vi "Machs.vi"(0 "Heizen?Mach1":bool, 1 "Heizen?Mach2":bool, 2 "PIDMach1":T1 {"proportional gain (Kc)" format="%.11g"; "integral gain (Kc*Ts/Ti)" format="%.11g"; "derivative gain (Kc*Td/Ts)" format="%.11g"}, 3 "PIDMach2":T1 {"proportional gain (Kc)" format="%.11g"; "integral gain (Kc*Ts/Ti)" format="%.11g"; "derivative gain (Kc*Td/Ts)" format="%.11g"}, 4 "Umax[V]Mach1":fxp<+/-,16,4> format="%.14g", 5 "Umax[V]Mach2":fxp<+/-,16,4> format="%.14g", 6 "USetp[V]Mach1":fxp<+/-,16,4> format="%.14g", 7 "USetp[V]Mach2":fxp<+/-,16,4> format="%.14g", 10 "Per[us]Mach":u16 caption="Periode Mach [us]", 11 "Mach1maxHigh":u16, 12 "vor der Messung [us]Mach":u16=200, 14 "wie viele Messwerte?Mach":u16, 15 "Mach2High?":bool, 16 "Abstand zwischen Messungen [us]Mach":u16 caption="Abstand zwischen Messungen Mach [us]", 17 "Mach2High":u16) -> (20 "U[V]Mach1":fxp<+/-,16,4> format="%.25g", 21 "U[V]Mach2":fxp<+/-,16,4> format="%.25g", 23 "Mach1maxHigh":u16, 26 "Mach2High?":bool, 27 "Mach2High":u16)   [LabVIEW 2010]
uses:
  <vilib>/eio/EIONode/EIONode.xnode
  <vilib>/rvi/eio/nirviEIOImplementation/nirviEIOImplementation.xnode
  <vilib>/rvi/eio/common/nirviEmuClasses.ctl
  <vilib>/rvi/FXPMathLib/FxpAdd/XNode/nifxpmath_Add.xnode
  <vilib>/rvi/FXPMathLib/FxpAdd/subVIs/nifxpmath_Add_SimConfig.ctl
  <vilib>/fxp/LVFixedPointQuantizationPolicyTypeDef.ctl
  <vilib>/fxp/LVFixedPointOverflowPolicyTypeDef.ctl
  <vilib>/rvi/FXPMathLib/FxpDiv/XNode/nifxpmath_Div.xnode
  <vilib>/rvi/FXPMathLib/FxpDiv/subVIs/nifxpmath_Div_SimConfig.ctl
  <vilib>/rvi/FXPMathLib/FxpMul/XNode/nifxpmath_Multiplier.xnode
  <vilib>/rvi/FXPMathLib/FxpMul/subVIs/nifxpmath_Mul_SimConfig.ctl
  <vilib>/rvi/FXPMathLib/FxpSqrt/XNode/nifxpmath_Sqrt.xnode
  <vilib>/rvi/FXPMathLib/FxpSqrt/subVIs/nifxpmath_Sqrt_SimConfig.ctl
  <vilib>/rvi/FXPMathLib/FxpConvert/XNode/nifxpmath_Convert.xnode
  <vilib>/rvi/FXPMathLib/FxpConvert/subVIs/nifxpmath_Convert_SimConfig.ctl
  <vilib>/addons/control/pid/fpga.llb/XNode/niFpgaPID.xnode
  <vilib>/rvi/eio/common/nirviEmuTemplateMethod_noerrors.vi
  <vilib>/rvi/FXPMathLib/FxpAdd/simVIs/DllFxpAddTemp_sub.vi
  <vilib>/rvi/FXPMathLib/FxpDiv/simVIs/DllFxpDivTemp_sub.vi
  <vilib>/rvi/FXPMathLib/FxpMul/simVIs/DllFxpMulTemp_sub.vi
  <vilib>/rvi/FXPMathLib/FxpSqrt/simVIs/DllSqrtTemp_sub.vi
  <vilib>/rvi/FXPMathLib/FxpConvert/simVIs/DllFxpConvertTemp_sub.vi
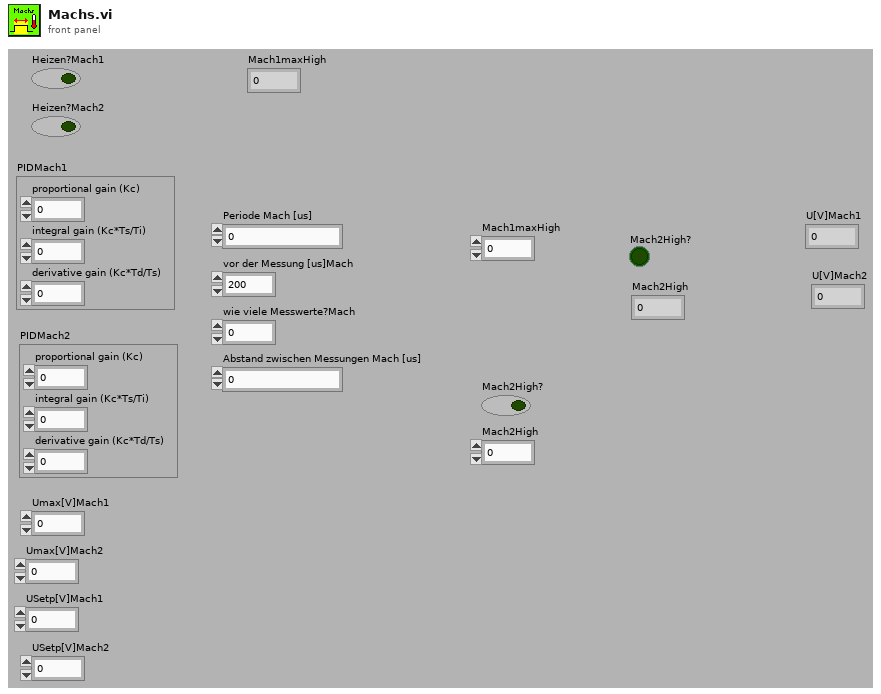
[diagram p1: front panel]
types:
  T1 = cluster{"proportional gain (Kc)":fxp<+/-,16,8>, "integral gain (Kc*Ts/Ti)":fxp<+/-,16,8>, "derivative gain (Kc*Td/Ts)":fxp<+/-,16,8>}
  T2 = cluster{"output high":fxp<+/-,16,4>, "output low":fxp<+/-,16,4>}
  T3 = typedef "nirviEmuClasses.ctl" = enum16{"IO Read", "IO Write", "Method", "Property Read", "Property Write"}
  T4 = cluster{"proportional gain (Kc)":i16, "integral gain (Kc*Ts/Ti)":i16, "derivative gain (Kc*Td/Ts)":i16}
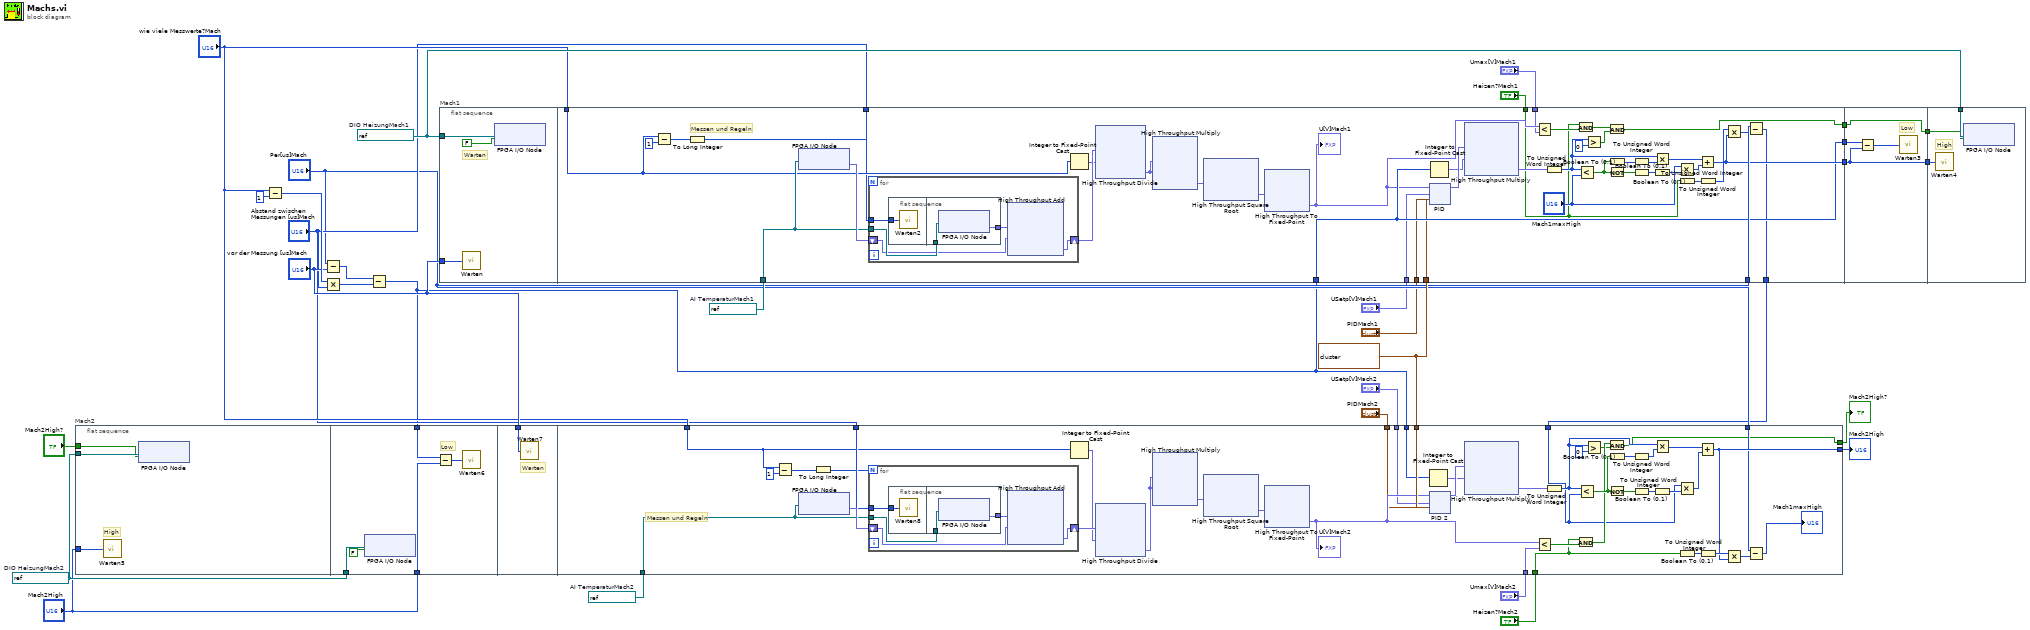
[diagram p0: block diagram]
diagram:
  w23 = refnum<k21> "Mod6/DIO22"  # DIO HeizungMach2
  w24 = refnum<k21> "Mod1/AI4"  # AI TemperaturMach2
  w25 = refnum<k21> "Mod1/AI3"  # AI TemperaturMach1
  w26 = refnum<k21> "Mod6/DIO23"  # DIO HeizungMach1
  w27 = T2 {"output high"=1.0, "output low"=0.0} ("output range")
  n1 = flat-sequence "Mach2" {
    tunnel: "Mach2High" -> [w33]
    tunnel: w23 -> [w35]
    tunnel: "Mach2High?" -> [w34]
    tunnel: w23 -> [w51]
    tunnel: w10 -> [w49]
    tunnel: "Mach2High" -> [w48]
    tunnel: "vor der Messung [us]Mach" -> [w63]
    tunnel: w24 -> [w104]
    tunnel: "Abstand zwischen Messungen [us]Mach" -> [w105]
    tunnel: "wie viele Messwerte?Mach" -> [w100]
    tunnel: w27 -> [w96]
    tunnel: w10 -> [w81]
    tunnel: [w82] -> w19
    tunnel: "Per[us]Mach" -> [w79]
    tunnel: [w74] -> w20
    tunnel: "USetp[V]Mach2" -> [w69]
    tunnel: "PIDMach2" -> [w68]
    tunnel: "Umax[V]Mach2" -> [w67]
    tunnel: "Heizen?Mach2" -> [w66]
    tunnel: w1 -> [w64]
    frame #0 {
      # "High"
      n2 = call "Warten5"("Count(uSec)"=w33) -> ()  [unwired: 1 out]
      n3 = xnode "FPGA I/O Node"("I/O Item"=w34, "FPGA I/O In"=w35) -> ()  [unwired: 1 out]
    }
    frame #1 {
      # "Low"
      n4 = xnode "FPGA I/O Node"("I/O Item"=FALSE, "FPGA I/O In"=w51) -> ()  [unwired: 1 out]
      n5 = Subtract(x=w49, y=w48) -> (x-y=w47:u16)
      n6 = call "Warten6"("Count(uSec)"=w47) -> ()  [unwired: 1 out]
    }
    frame #2 {
      # "Warten"
      n7 = call "Warten7"("Count(uSec)"=w63) -> ()  [unwired: 1 out]
    }
    frame #3 {
      # "Messen und Regeln"
      n8 = Subtract(x=w100, y=u16 1) -> (x-y=w102:u16)
      n9 = xnode "FPGA I/O Node"("FPGA I/O In"=w104) -> ("I/O Item"=w106:fxp<+/-,26,5>)  [unwired: 1 out]
      n10 = To Long Integer(number=w102) -> (32bit integer=w101:i32)
      n11 = for {
        N: w101 -> [_]
        shift-right: [w274] -> w99
        shift-left: w106 -> [w275]
        tunnel: w105 -> [w278]
        tunnel: w104 -> [w277]
        n12 = flat-sequence {
          tunnel: w278 -> [w309]
          tunnel: w277 -> [w311]
          tunnel: [w310] -> w276
          frame #0 {
            n13 = call "Warten8"("Count(uSec)"=w309) -> ()  [unwired: 1 out]
          }
          frame #1 {
            n14 = xnode "FPGA I/O Node"("FPGA I/O In"=w311) -> ("I/O Item"=w310:fxp<+/-,26,5>)  [unwired: 1 out]
          }
        }
        n15 = xnode "High Throughput Add"("x"=w276, "y"=w275) -> ("x+y"=w274:fxp<+/-,32,11>)
      }
      n16 = Integer to Fixed-Point Cast ("Integer in Festkomma umwandeln")(integer=w100) -> (fixed-point=w98:fxp<+/-,8,8>)  [unwired: 1 in]
      n17 = xnode "High Throughput Divide"("x"=w99, "y"=w98) -> ("x/y"=w73:fxp<+/-,16,4>)
      n18 = xnode "High Throughput Multiply"("x"=w73, "y"=w73) -> ("x*y"=w72:fxp<+,32,8>)
      n19 = xnode "High Throughput Square Root"("x"=w72) -> ("sqrt(x)"=w71:fxp<+,16,4>)
      n20 = xnode "High Throughput To Fixed-Point"("x"=w71) -> ("y"=w70:fxp<+/-,16,4>)
      "U[V]Mach2" <- w70
      n21 = xnode ("PID 2")("process variable"=w70, "setpoint"=w69, "PID gains"=w68, "output range"=w96) -> ("output"=w95:fxp<+/-,16,4>)  [unwired: 1 in]
      n22 = Integer to Fixed-Point Cast ("Integer in Festkomma umwandeln")(integer=w81) -> (fixed-point=w94:fxp<+,16,16>)  [unwired: 1 in]
      n23 = xnode "High Throughput Multiply"("x"=w95, "y"=w94) -> ("x*y"=w85:fxp<+/-,16,16>)
      n24 = Less?(x=w70, y=w67) -> (x < y?=w97:bool)
      n25 = To Unsigned Word Integer(number=w85) -> (unsigned 16bit integer=w77:u16)
      n26 = And(x=w66, y=w97) -> (x .and. y?=w76:bool)
      n27 = Less?(x=w77, y=w64) -> (x < y?=w89:bool)
      n28 = Greater?(x=w77, y=u16 0) -> (0:w75:bool)
      n29 = And(x=w76, y=w75) -> (x .and. y?=w74:bool)
      n30 = Boolean To (0,1)(Boolean=w89) -> (0, 1=w93:i16)
      n31 = Not(x=w89) -> (.not. x?=w88:bool)
      n32 = To Unsigned Word Integer(number=w93) -> (unsigned 16bit integer=w92:u16)
      n33 = Boolean To (0,1)(Boolean=w88) -> (0, 1=w91:i16)
      n34 = Multiply(x=w77, y=w92) -> (x*y=w87:u16)
      n35 = To Unsigned Word Integer(number=w91) -> (unsigned 16bit integer=w90:u16)
      n36 = Multiply(x=w64, y=w90) -> (x*y=w86:u16)
      n37 = Boolean To (0,1)(Boolean=w66) -> (0, 1=w84:i16)
      n38 = Add(x=w87, y=w86) -> (x+y=w82:u16)
      n39 = To Unsigned Word Integer(number=w84) -> (unsigned 16bit integer=w83:u16)
      n40 = Multiply(x=w83, y=w82) -> (x*y=w80:u16)
      n41 = Subtract(x=w79, y=w80) -> (x-y=→"Mach1maxHigh":u16)
    }
  }
  n42 = Subtract(x="wie viele Messwerte?Mach", y=u16 1) -> (x-y=w17:u16)
  n43 = Subtract(x="Per[us]Mach", y="vor der Messung [us]Mach") -> (x-y=w16:u16)
  n44 = Multiply(x=w17, y="Abstand zwischen Messungen [us]Mach") -> (x*y=w15:u16)
  n45 = Subtract(x=w16, y=w15) -> (x-y=w10:u16)
  n46 = flat-sequence "Mach1" {
    tunnel: "vor der Messung [us]Mach" -> [w352]
    tunnel: w26 -> [w351]
    tunnel: w25 -> [w404]
    tunnel: "Abstand zwischen Messungen [us]Mach" -> [w400]
    tunnel: "wie viele Messwerte?Mach" -> [w402]
    tunnel: "Per[us]Mach" -> [w385]
    tunnel: [w376] -> w32
    tunnel: [w379] -> w31
    tunnel: [w374] -> w30
    tunnel: w10 -> [w374]
    tunnel: w27 -> [w373]
    tunnel: "Umax[V]Mach1" -> [w368]
    tunnel: "USetp[V]Mach1" -> [w367]
    tunnel: "Heizen?Mach1" -> [w366]
    tunnel: "PIDMach1" -> [w365]
    tunnel: [w364] -> w1
    tunnel: [w652] -> w29
    tunnel: w32 -> [w652]
    tunnel: [w653] -> w28
    tunnel: w31 -> [w653]
    tunnel: w30 -> [w651]
    tunnel: w26 -> [w656]
    tunnel: w29 -> [w655]
    tunnel: w28 -> [w654]
    frame #0 {
      # "Warten"
      n47 = call "Warten"("Count(uSec)"=w352) -> ()  [unwired: 1 out]
      n48 = xnode "FPGA I/O Node"("I/O Item"=FALSE, "FPGA I/O In"=w351) -> ()  [unwired: 1 out]
    }
    frame #1 {
      # "Messen und Regeln"
      n49 = Subtract(x=w402, y=u16 1) -> (x-y=w399:u16)
      n50 = To Long Integer(number=w399) -> (32bit integer=w398:i32)
      n51 = xnode "FPGA I/O Node"("FPGA I/O In"=w404) -> ("I/O Item"=w406:fxp<+/-,26,5>)  [unwired: 1 out]
      n52 = for {
        N: w398 -> [_]
        shift-right: [w547] -> w403
        shift-left: w406 -> [w548]
        tunnel: w400 -> [w551]
        tunnel: w404 -> [w550]
        n53 = flat-sequence {
          tunnel: w551 -> [w582]
          tunnel: w550 -> [w584]
          tunnel: [w583] -> w549
          frame #0 {
            n54 = call "Warten2"("Count(uSec)"=w582) -> ()  [unwired: 1 out]
          }
          frame #1 {
            n55 = xnode "FPGA I/O Node"("FPGA I/O In"=w584) -> ("I/O Item"=w583:fxp<+/-,26,5>)  [unwired: 1 out]
          }
        }
        n56 = xnode "High Throughput Add"("x"=w549, "y"=w548) -> ("x+y"=w547:fxp<+/-,32,11>)
      }
      n57 = Integer to Fixed-Point Cast ("Integer in Festkomma umwandeln")(integer=w402) -> (fixed-point=w401:fxp<+/-,8,8>)  [unwired: 1 in]
      n58 = xnode "High Throughput Divide"("x"=w403, "y"=w401) -> ("x/y"=w372:fxp<+/-,16,4>)
      n59 = xnode "High Throughput Multiply"("x"=w372, "y"=w372) -> ("x*y"=w371:fxp<+,32,8>)
      n60 = xnode "High Throughput Square Root"("x"=w371) -> ("sqrt(x)"=w370:fxp<+,16,4>)
      n61 = xnode "High Throughput To Fixed-Point"("x"=w370) -> ("y"=w369:fxp<+/-,16,4>)
      "U[V]Mach1" <- w369
      n62 = xnode ("PID")("process variable"=w369, "setpoint"=w367, "PID gains"=w365, "output range"=w373) -> ("output"=w397:fxp<+/-,16,4>)  [unwired: 1 in]
      n63 = Integer to Fixed-Point Cast ("Integer in Festkomma umwandeln")(integer=w374) -> (fixed-point=w396:fxp<+,16,16>)  [unwired: 1 in]
      n64 = xnode "High Throughput Multiply"("x"=w397, "y"=w396) -> ("x*y"=w395:fxp<+/-,16,16>)
      n65 = Less?(x=w369, y=w368) -> (x < y?=w384:bool)
      n66 = To Unsigned Word Integer(number=w395) -> (unsigned 16bit integer=w383:u16)
      n67 = And(x=w366, y=w384) -> (x .and. y?=w381:bool)
      n68 = Less?(x=w383, y="Mach1maxHigh") -> (x < y?=w390:bool)
      n69 = Greater?(x=w383, y=u16 0) -> (0:w380:bool)
      n70 = And(x=w381, y=w380) -> (x .and. y?=w379:bool)
      n71 = Boolean To (0,1)(Boolean=w390) -> (0, 1=w394:i16)
      n72 = Not(x=w390) -> (.not. x?=w389:bool)
      n73 = To Unsigned Word Integer(number=w394) -> (unsigned 16bit integer=w393:u16)
      n74 = Boolean To (0,1)(Boolean=w389) -> (0, 1=w392:i16)
      n75 = Multiply(x=w383, y=w393) -> (x*y=w387:u16)
      n76 = To Unsigned Word Integer(number=w392) -> (unsigned 16bit integer=w391:u16)
      n77 = Multiply(x="Mach1maxHigh", y=w391) -> (x*y=w386:u16)
      n78 = Boolean To (0,1)(Boolean=w366) -> (0, 1=w378:i16)
      n79 = Add(x=w387, y=w386) -> (x+y=w376:u16)
      n80 = To Unsigned Word Integer(number=w378) -> (unsigned 16bit integer=w377:u16)
      n81 = Multiply(x=w377, y=w376) -> (x*y=w375:u16)
      n82 = Subtract(x=w385, y=w375) -> (x-y=w364:u16)
    }
    frame #2 {
      # "Low"
      n83 = Subtract(x=w651, y=w652) -> (x-y=w650:u16)
      n84 = call "Warten3"("Count(uSec)"=w650) -> ()  [unwired: 1 out]
    }
    frame #3 {
      # "High"
      n85 = call "Warten4"("Count(uSec)"=w655) -> ()  [unwired: 1 out]
      n86 = xnode "FPGA I/O Node"("I/O Item"=w654, "FPGA I/O In"=w656) -> ()  [unwired: 1 out]
    }
  }
  "Mach2High?" <- w20
  "Mach2High" <- w19
